vi "error handler.vi"(8 "error in (no error)":errorcluster, 11 "Next State In":T1) -> (0 "error out":errorcluster, 3 "Next State Out":T1)   [LabVIEW 2013]
uses:
  Electrical Measurements/Controls/StateMachineStates.ctl
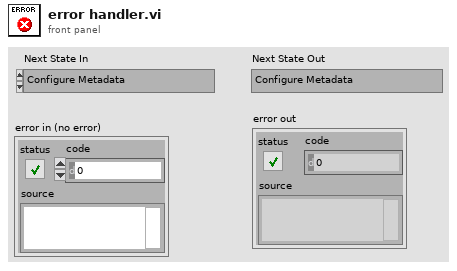
[diagram p1: front panel]
types:
  T1 = typedef "StateMachineStates.ctl" = enum16{"Configure Metadata", "Initialize", "Idle", "Calibration", "Aux Correction", "Stabilize", "Take Measurement", "Write Data", "Check If Data is Good", "Write Flicker Dark", "Notify Operator", "Stop"}
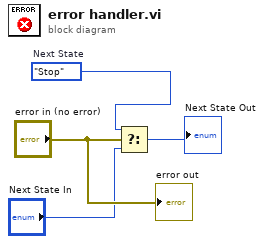
[diagram p0: block diagram]
diagram:
  w3 = StateMachineStates."Stop"  # Next State
  n1 = Select(t=w3, s="error in (no error)", f="Next State In") -> (s? t:f=→"Next State Out":T1)
  "error out" <- "error in (no error)"
